vi "Rotate Radians.vi"(0 "Radians to turn(Direction)":dbl format="%#_13g", 5 "Swerve DevRef":T1[](array[typedef]), 7 "Wheel DevRef":T1[](array[typedef]), 11 "error in":errorcluster) -> (15 "error constant":errorcluster)   [LabVIEW 2016]
uses:
  <vilib>/Rock Robotics/SystemInterfaces/DIO/FPGA_DIOPWMChannel.ctl
  <vilib>/Rock Robotics/WPI/PWM/WPI_PWMDeadband.ctl
  <vilib>/Rock Robotics/WPI/MotorControl/WPI_MotorControlType.ctl
  <vilib>/Rock Robotics/WPI/MotorControl/WPI_MotorControlDeviceRef.ctl
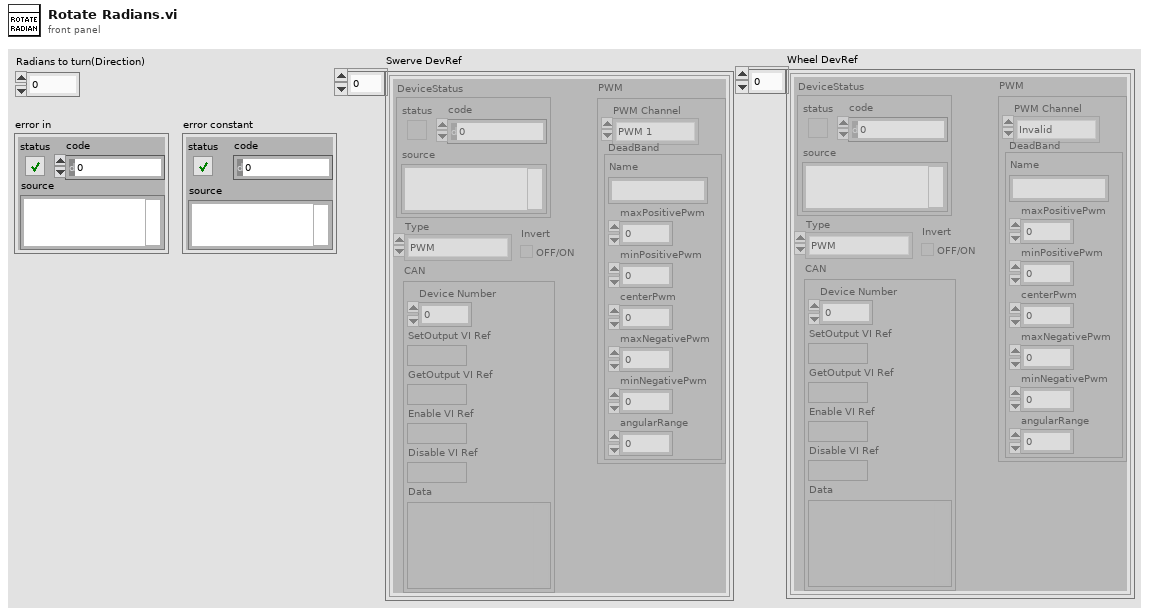
[diagram p1: front panel]
types:
  T1 = typedef "WPI_MotorControlDeviceRef.ctl" = cluster{"DeviceStatus":errorcluster, "Type":T2, "PWM":cluster{"PWM Channel":T3, "DeadBand":T4}, "CAN":cluster{"Device Number":u8, "SetOutput VI Ref":variant, "GetOutput VI Ref":variant, "Enable VI Ref":variant, "Disable VI Ref":variant, "Data":variant}, "Invert":bool}
  T2 = typedef "WPI_MotorControlType.ctl" = enum16{"PWM", "CAN"}
  T3 = typedef "FPGA_DIOPWMChannel.ctl" = enum8{"PWM 0", "PWM 1", "PWM 2", "PWM 3", "PWM 4", "PWM 5", "PWM 6", "PWM 7", "PWM 8", "PWM 9", "PWM MXP 0", "PWM MXP 1", "PWM MXP 2", "PWM MXP 3", "PWM MXP 4", "PWM MXP 5", "PWM MXP 6", "PWM MXP 7", "PWM MXP 8", "PWM MXP 9", "Invalid"}
  T4 = typedef "WPI_PWMDeadband.ctl" = cluster{"Name":string, "maxPositivePwm":i32, "minPositivePwm":i32, "centerPwm":i32, "maxNegativePwm":i32, "minNegativePwm":i32, "angularRange":u16}
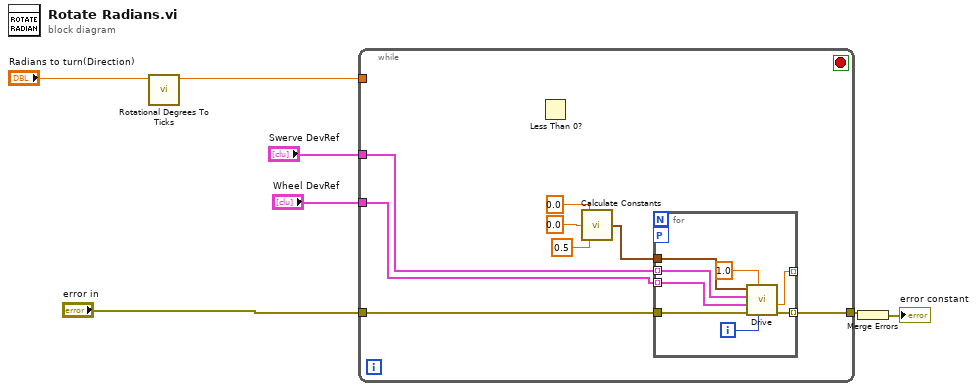
[diagram p0: block diagram]
diagram:
  n1 = call "Rotational Degrees To Ticks.vi"("Rotational Degrees"="Radians to turn(Direction)") -> ("Ticks"=w1:dbl)  [unwired: 10 in]
  n2 = while {
    tunnel: w1 -> [_]
    tunnel: "Swerve DevRef" -> [w14]
    tunnel: "Wheel DevRef" -> [w13]
    tunnel: "error in" -> [w9]
    tunnel: [w12] -> w3
    stop <- _ stop-if-true
    n3 = Less Than 0?() -> ()  [unwired: 1 in, 1 out]
    n4 = call "Calculate Constants.vi"("Z"=0.5, "Y"=0.0, "X"=0.0) -> ("constants cluster"=w11:cluster{"a":dbl, "b":dbl, "c":dbl, "d":dbl})
    n5 = for {
      tunnel: w11 -> [w23]
      tunnel: w14 -> [w22] mode=indexing
      tunnel: w13 -> [w21] mode=indexing
      tunnel: w9 -> [w19]
      tunnel: [w18] -> w12 mode=indexing
      workers-P: _ -> [_]
      tunnel: [w16] -> _ mode=indexing
      i -> [w17]
      n6 = call "Drive.vi"("Index"=w17, "Max Speed or 1"=1.0, "error in"=w19, "Wheel DevRef"=w21, "Swerve DevRef"=w22, "constants"=w23) -> ("error out"=w18:errorcluster, "Wheel Speed"=w16:dbl)  [unwired: 1 in, 3 out]
    }
  }
  n7 = Merge Errors(w3) -> (→"error constant":errorcluster)
